vi "End Report.vi"(8 "error in (no error)":errorcluster {"code" format="Error %.0f"}, 11 "VIDoc Printer In":refnum<class "VIDoc Printer.lvclass">) -> (0 "error out":errorcluster {"code" format="Error %.0f"}, 3 "VIDoc Printer Out":refnum<class "VIDoc Printer.lvclass">)   [LabVIEW 2023, in "VIDoc Printer.lvlib" / "VIDoc Printer.lvclass"]
uses:
  VIDoc Printer.lvclass
  VIDoc Printer.lvclass/VIDoc Printer.ctl
  UI Interaction/Interface/UI Interaction.lvclass
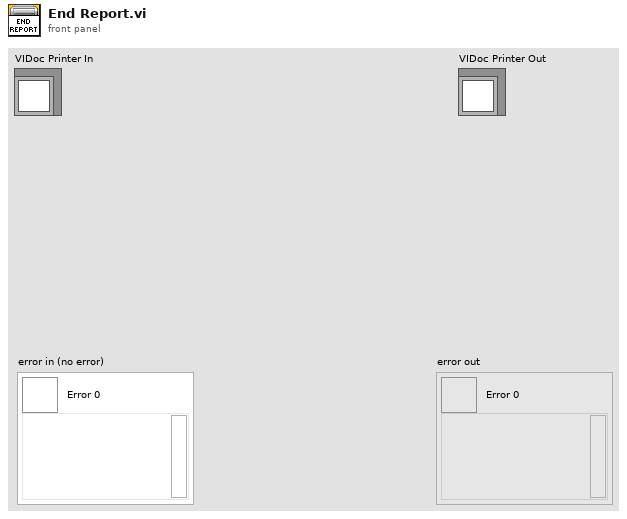
[diagram p1: front panel]
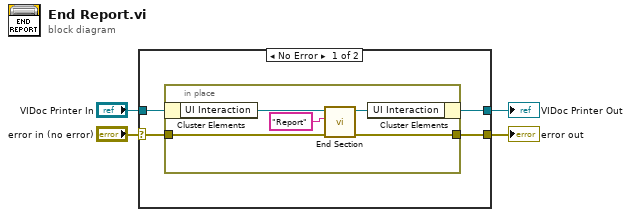
[diagram p0: block diagram]
diagram:
  n1 = case shown="No Error" "error in (no error)" {
    selector: "error in (no error)" -> [w7 w15]
    tunnel: [w6 w15] -> w3
    tunnel: [w8 w14] -> w1
    tunnel: "VIDoc Printer In" -> [w5 w14]
    frame No Error {
      n2 = in-place {
        in-place-border: w7 -> [w11]
        in-place-border: [w10] -> w6
        n3 = in-place-cluster #1(w5) -> ("UI Interaction"=w13:refnum<class "UI Interaction.lvclass">)
        n4 = call-dynamic "End Section.vi"("error in (no error)"=w11, "Section"="Report", "UI Interaction in"=w13) -> ("error out"=w10:errorcluster, "UI Interaction out"=w12:refnum<class "UI Interaction.lvclass">)  [unwired: 7 in]
        n5 = in-place-cluster #1("UI Interaction"=w12) -> (w8:refnum<class "VIDoc Printer.lvclass">)
      }
    }
    frame Error {
    }
  }
  "error out" <- w3
  "VIDoc Printer Out" <- w1
